vi "Decode TextString.vi"(11 "Length-Prefixed Field":u8[](array[numeric]) format="%08b") -> (2 "Text String":string, 3 "Remaining Packets":u8[](array[numeric]) format="%08b")   [LabVIEW 2013, in "ControlPacket.lvclass"]
uses:
  ControlPacket.lvclass
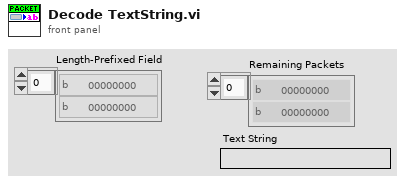
[diagram p1: front panel]
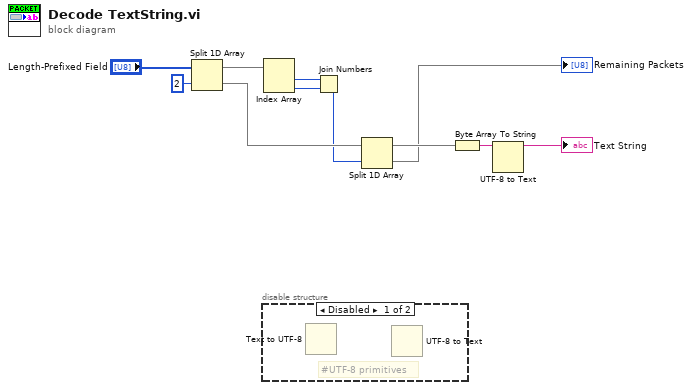
[diagram p0: block diagram]
diagram:
  n1 = Split 1D Array(array="Length-Prefixed Field", index=2) -> (first subarray=w10:u8[], second subarray=w8:u8[])
  n2 = disable-structure shown="Disabled" {
    frame Disabled {
      # "#UTF-8 primitives"
      n3 = Text to UTF-8() -> ()  [unwired: 2 in, 2 out]
      n4 = UTF-8 to Text() -> ()  [unwired: 2 in, 2 out]
    }
    frame Enabled {
    }
  }
  n5 = Index Array(array=w10) -> (element #1=w3:u8, element #2=w4:u8)  [unwired: 2 in]
  n6 = Join Numbers(hi=w3, lo=w4) -> ((hi.lo)=w2:u16)
  n7 = Split 1D Array(array=w8, index=w2) -> (first subarray=w7:u8[], second subarray=→"Remaining Packets":u8[])
  n8 = Byte Array To String(unsigned byte array=w7) -> (string=w9:string)
  n9 = UTF-8 to Text(11:w9) -> (3:→"Text String":string)  [unwired: 1 in, 1 out]
